vi "FRC Color Processing Example.vi"() -> ()   [LabVIEW 2019]
uses:
  <vilib>/Rock Robotics/WPI/Camera/WPI_CameraSettings Read MJPG.ctl
  <vilib>/Rock Robotics/WPI/Camera/WPI_CameraImageSize.ctl
  Vision Support Code/Camera Types.ctl
  <vilib>/Rock Robotics/WPI/Camera/WPI_CameraExposure Values.ctl
  <vilib>/Rock Robotics/WPI/Camera/WPI_CameraWhite Balance Values.ctl
  <vilib>/vision/NI_Vision_Development_Module.lvlib
panel:
  out "Number of Particles":i32
  out "Particle Measurements (Pixels)":dbl[][](array[numeric]) format="%.2f"
  out "Particle Measurements (Real-World)":dbl[][](array[numeric]) format="%.2f"
  in  "Min Compnt %":dbl=15.0
  out "Results":T1(array[cluster]) {"Score" format="%#_3g"; "Pixels"."Rectangle"."Numeric 5" format="%#_3g"; "Pixels"."Rectangle"."Numeric 3" format="%#_3g"; "Pixels"."Rectangle"."Numeric 2" format="%#_3g"; "Pixels"."Rectangle"."Numeric" format="%#_3g"; "Normalized"."Rectangle"."Numeric 5" format="%#_2g"; "Normalized"."Rectangle"."Numeric 3" format="%#_2g"; "Normalized"."Rectangle"."Numeric 2" format="%#_2g"; "Normalized"."Rectangle"."Numeric" format="%#_2g"; "Normalized"."Center"."?" format="%#_3g"; "Normalized"."Center"."?" format="%#_3g"; "Distance (ft)" format="%#_3g"}
  in  "Size Limit %":dbl=0.04 min=0.0 max=100.0 step=0.01 format="%#_13g"
  out "Instructions:":string="Instructions:\nUse Source to load image files from a directory, or use a USB or IP camera connected to your laptop. Use Camera Settings 1 and 2 to achieve a dark image with bright and colorful stripes.\nLED Color can encoded as HSL or related color modes. Calibrate to the same color as the strips being reflected to the camera.\nClick and draw a line in Original Image to auto-calibrate the LED Color. You may want to widen and tweak Sat and Val by hand.\nThe Annotate button affects drawing a rectangle around the stripes and labeling it with a distance in ft. Distance relies on knowing the Camera Type and lens calibration (it looks up the lens view angle).\n\nAdjust Score Cutoff to make the code more or less picky. If the color is not very unique, you may need to increase the number of particles considered. The diagram uses a Size Limit to ignore colored things that are too small. You may need to adjust it if you are targetting from far away.\n\nResults give you the distance to the target, the center and box in a normalized (-1 to 1) and pixel coordinates.\n\nBe sure to read about setting camera exposure and brightness to help simplify your image and acquire color saturated images.\n\nThere are lots of comments on the diagram to explain the code."
  in  "Color Mode":u16(ring)=2 items=["RGB", "HSL", "HSV", "HSI"]
  in  "Particles":dbl=5.0
  in  "Score Cutoff %":dbl=75.0
  in  "Std Devs for Calibration":cluster{"H":dbl, "S":dbl, "V":dbl}={"H"=4.0, "S"=8.0, "V"=8.0}
  in  "Camera Type (for distance)":T2=enum."MS HD3000 square"
  in  "image files":string[](array[string])
  in  "Source":enum32{"Files", "Camera"}(tab)
  in  "Images":i32(listbox)
  in  "Folder Location":path=path "C:/Program Files (x86)/National Instruments/LabVIEW 2018/examples/FRC/roboRIO/Vision/2019 Vision Example/Sample Images"
  in  "Camera Settings":T3={"fps"=20, "compression"=30, "Image Size"=enum."320x240", "Config Shown"=FALSE}
  in  "Camera Address":string="USB 1"
  in  "Camera Settings 2":T7={"Exposure"=enum."Auto", "Exposure (%)"=50.0, "Brightness"=50, "White Balance"=enum."Auto", "Color Temp (K)"=0.0} {"Brightness" min=0 max=100}
  in  "Annotate":bool=TRUE
  out "Qualified Particles":i32
  in  "LED Color Range":T8={"Hue"={75.46666717529297, 107.46666717529297}, "Sat"={221.18788146972656, 255.0}, "Val"={23.733230590820312, 172.13343811035156}} {"Hue" scale=0.0..255.0 scale format="%#_3g"}
  out "Mask":T9(plugin-control)
  out "Original Image":T9(plugin-control)
  # "Good target rectangle, distance ft"
  # "Bad target rectangle"
  # "Score in %"
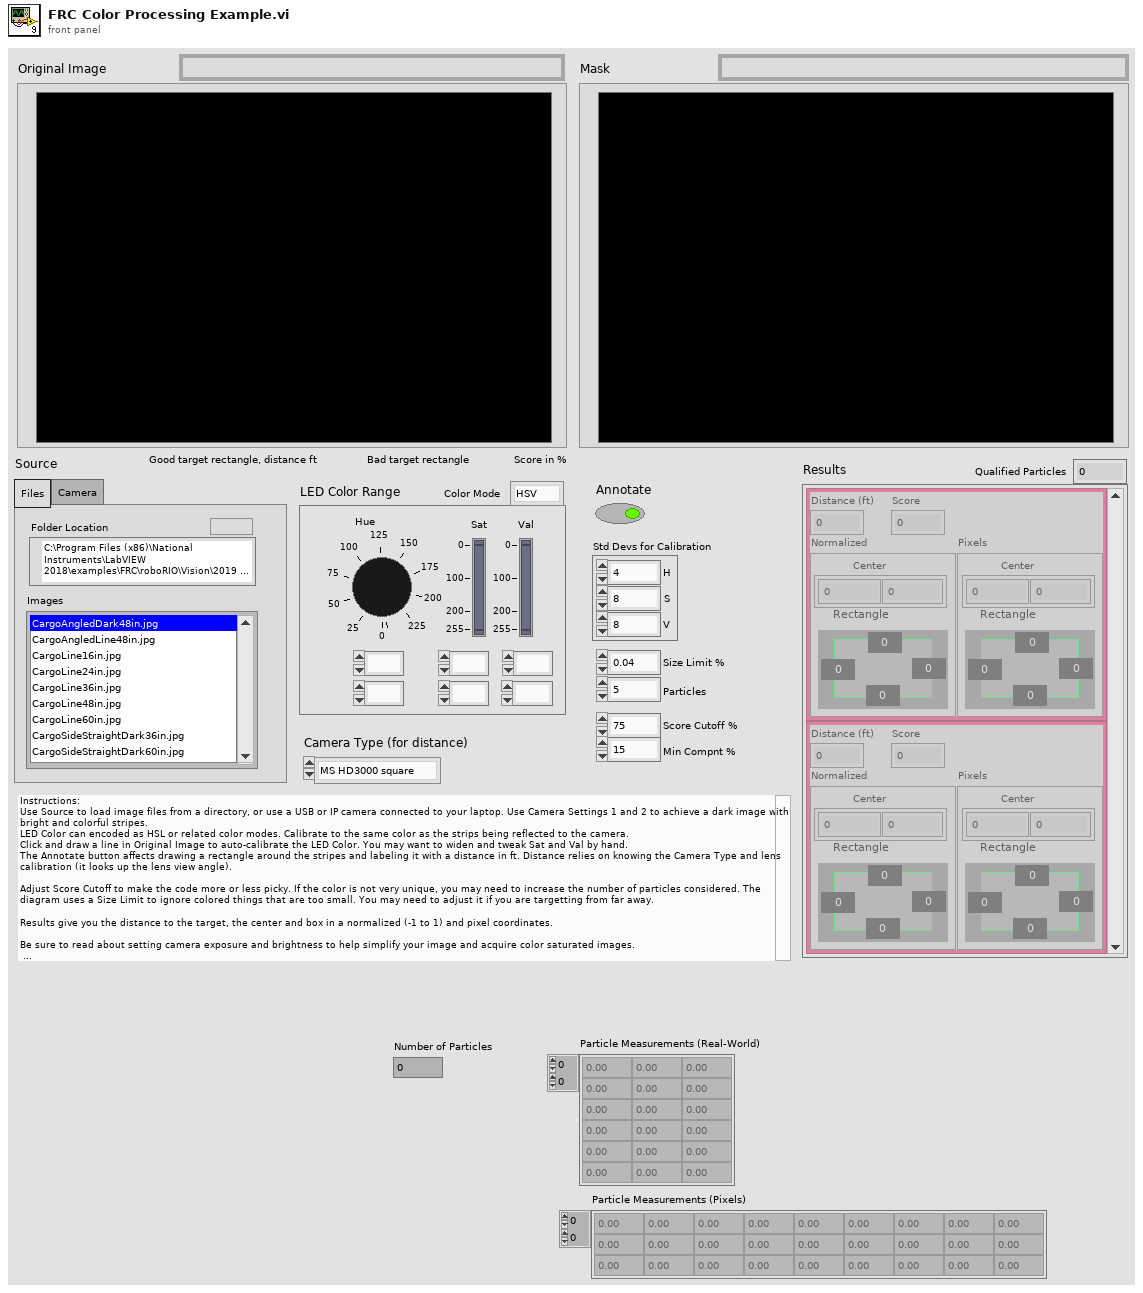
[diagram p1: front panel]
types:
  T1 = cluster{"Distance (ft)":dbl, "Score":dbl, "Normalized":cluster{"Center":cluster{dbl, dbl}, "Rectangle":cluster{"Numeric":dbl, "Numeric 2":dbl, "Numeric 3":dbl, "Numeric 5":dbl}}, "Pixels":cluster{"Center":cluster{dbl, dbl}, "Rectangle":cluster{"Numeric":dbl, "Numeric 2":dbl, "Numeric 3":dbl, "Numeric 5":dbl}}}[]
  T2 = typedef "Camera Types.ctl" = enum16{"206", "1011", "1013", "MS HD3000 square", "MS HD3000 640x480"}
  T3 = typedef "WPI_CameraSettings Read MJPG.ctl" = cluster{"fps":i32, "compression":i32, "Image Size":T4, "Config Shown":bool}
  T4 = typedef "WPI_CameraImageSize.ctl" = enum16{"640x480", "320x240", "160x120", "Custom"}
  T5 = typedef "WPI_CameraExposure Values.ctl" = enum16{"Auto", "Flicker-free 50 Hz", "Flicker-free 60 Hz", "Hold current", "Custom"}
  T6 = typedef "WPI_CameraWhite Balance Values.ctl" = enum16{"Auto", "Fixed indoor", "Fixed outdoor 1", "Fixed outdoor 2", "Fixed fluorescent 1", "Fixed fluorescent 2", "Hold current", "Custom"}
  T7 = cluster{"Exposure":T5, "Exposure (%)":dbl, "Brightness":i32, "White Balance":T6, "Color Temp (K)":dbl}
  T8 = cluster{"Hue":cluster{dbl, dbl}, "Sat":cluster{dbl, dbl}, "Val":cluster{dbl, dbl}}
  T9 = typedef "IMAQ Image.ctl" = refnum<image>
  T10 = typedef "Particle Parameters" = i32
  T11 = typedef "Image Type" = u32
  T12 = cluster{cluster{dbl, dbl}, cluster{dbl, dbl}, cluster{dbl, dbl}}
  T13 = cluster{"Score":dbl, "Rect":cluster{"Left":dbl, "Top":dbl, "Right":dbl, "Bottom":dbl}, "Full Scores":cluster{"Aspect Ratio":dbl, "Top Position":dbl, "Bottom Position":dbl, "Left Gap":dbl, "Width":dbl, "Height Ratio":dbl, "Angle":dbl}}[]
  T14 = cluster{"Left":dbl, "Top":dbl, "Right":dbl, "Bottom":dbl}
  T15 = cluster{"Distance (ft)":dbl, "Score":dbl, "Normalized":cluster{"Center":cluster{dbl, dbl}, "Rectangle":cluster{"Numeric":dbl, "Numeric 2":dbl, "Numeric 3":dbl, "Numeric 5":dbl}}, "Pixels":cluster{"Center":cluster{dbl, dbl}, "Rectangle":cluster{"Numeric":dbl, "Numeric 2":dbl, "Numeric 3":dbl, "Numeric 5":dbl}}}
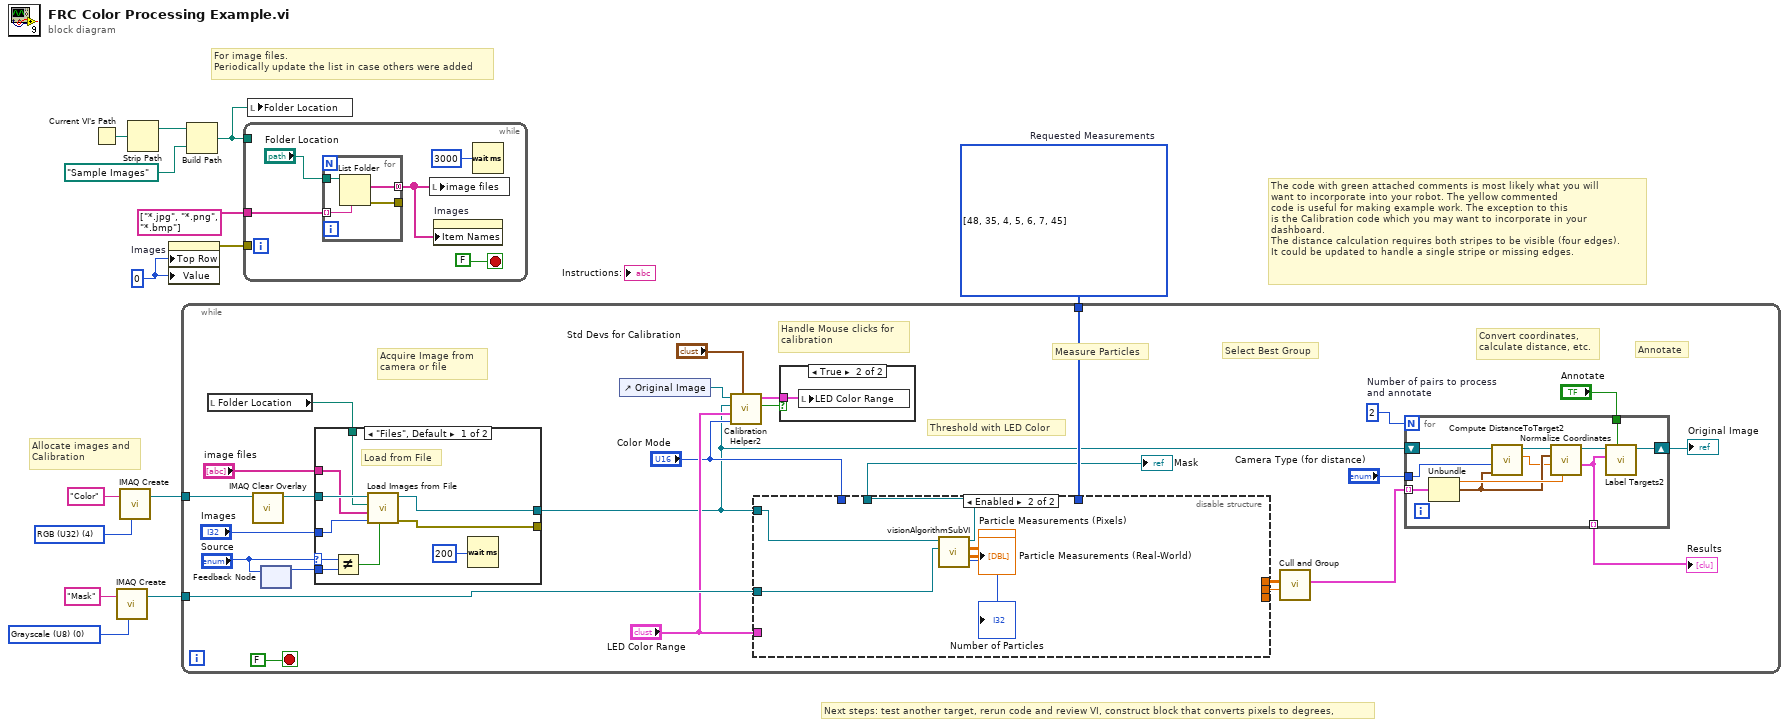
[diagram p0: block diagram]
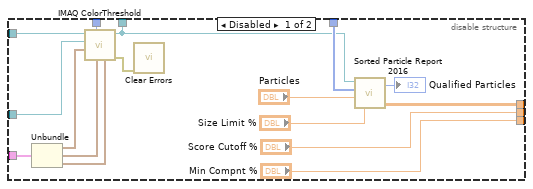
[diagram p2: hidden frame]
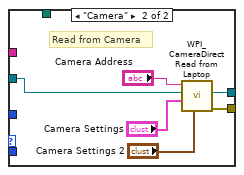
[diagram p4: hidden frame]
diagram:
  w3 = u32 0 ("milliseconds to wait")
  w9 = T10[] [48, 35, 4, 5, 6, 7, 45] items=["Center of Mass X", "Center of Mass Y", "First Pixel X", "First Pixel Y", "Bounding Rect Left", "Bounding Rect Top", "Bounding Rect Right", "Bounding Rect Bottom", "Max Feret Diameter Start X", "Max Feret Diameter Start Y", "Max Feret Diameter End X", "Max Feret Diameter End Y", "Max Horiz. Segment Length Left", "Max Horiz. Segment Length Right", "Max Horiz. Segment Length Row", "-", "Bounding Rect Width", "Bounding Rect Height", "Bounding Rect Diagonal", "Perimeter", "Convex Hull Perimeter", "Holes' Perimeter", "Max Feret Diameter", "Equivalent Ellipse Major Axis", "Equivalent Ellipse Minor Axis", "Equivalent Ellipse Minor Axis (Feret)", "Equivalent Rect Long Side", "Equivalent Rect Short Side", "Equivalent Rect Diagonal", "Equivalent Rect Short Side (Feret)", "Average Horiz. Segment Length", "Average Vert. Segment Length", "Hydraulic Radius", "Waddel Disk Diameter", "-", "Area", "Holes' Area", "Particle & Holes' Area", "Convex Hull Area", "Image Area", "-", "Number of Holes", "Number of Horiz. Segments", "Number of Vert. Segments", "-", "Orientation", "Max Feret Diameter Orientation", "-", "% Area/Image Area", "% Area/(Particle & Holes' Area)", "Ratio of Equivalent Ellipse Axes", "Ratio of Equivalent Rect Sides", "-", "Elongation Factor", "Compactness Factor", "Heywood Circularity Factor", "Type Factor", "-", "Sum X", "Sum Y", "Sum XX", "Sum XY", "Sum YY", "Sum XXX", "Sum XXY", "Sum XYY", "Sum YYY", "-", "Moment of Inertia XX", "Moment of Inertia XY", "Moment of Inertia YY", "Moment of Inertia XXX", "Moment of Inertia XXY", "Moment of Inertia XYY", "Moment of Inertia YYY", "Norm. Moment of Inertia XX", "Norm. Moment of Inertia XY", "Norm. Moment of Inertia YY", "Norm. Moment of Inertia XXX", "Norm. Moment of Inertia XXY", "Norm. Moment of Inertia XYY", "Norm. Moment of Inertia YYY", "Hu Moment 1", "Hu Moment 2", "Hu Moment 3", "Hu Moment 4", "Hu Moment 5", "Hu Moment 6", "Hu Moment 7"]  # Requested Measurements
  w12 = T11 0 items=["Grayscale (U8)", "Grayscale (I16)", "Grayscale (SGL)", "Complex (CSG)", "RGB (U32)", "HSL (U32)", "RGB (U64)", "Grayscale (U16)"] ("Image Type")
  w13 = T11 4 items=["Grayscale (U8)", "Grayscale (I16)", "Grayscale (SGL)", "Complex (CSG)", "RGB (U32)", "HSL (U32)", "RGB (U64)", "Grayscale (U16)"] ("Image Type")
  # "Next steps: test another target, rerun code and review VI, construct block that converts pixels to degrees,"
  # "The code with green attached comments is most likely what you will\nwant to incorporate into your robot. The yellow commented\ncode is useful for making example work. The exception to this\nis the Calibration code which you may want to incorporate in your\ndashboard.\nThe distance calculation requires both stripes to be visible (four edges).\nIt could be updated to handle a single stripe or missing edges."
  # "For image files.\nPeriodically update the list in case others were added"
  # "Allocate images and\nCalibration"
  n1 = Current VI's Path() -> (path=w8:path)
  n2 = call "IMAQ Create"("Image Name"="Mask", "Image Type"=w12) -> ("New Image"=w10:T9)  [unwired: 2 in, 2 out]
  n3 = call "IMAQ Create"("Image Name"="Color", "Image Type"=w13) -> ("New Image"=w1:T9)  [unwired: 2 in, 2 out]
  n4 = Strip Path(path=w8) -> (stripped path=w6:path)  [unwired: 1 out]
  n5 = property on="Images" class="LstBox (strict)"("Top Row"=w3, "Value"=w3) -> (error out=w4:errorcluster)  [unwired: 2 in, 1 out]
  n6 = while {
    tunnel: w1 -> [w20]
    tunnel: w10 -> [w38]
    tunnel: w9 -> [w37]
    stop <- FALSE stop-if-true
    w21 = 2  # Number of pairs to process and annotate
    # "Handle Mouse clicks for\ncalibration"
    # "Measure Particles"
    # "Convert coordinates,\ncalculate distance, etc."
    # "Annotate"
    # "Select Best Group"
    # "Threshold with LED Color"
    # "Acquire Image from\ncamera or file"
    n7 = local read "Folder Location"() -> (w30:path)
    n8 = call "IMAQ Clear Overlay"("Image"=w20) -> ("Image Out"=w19:T9)  [unwired: 2 in, 8 out]
    n9 = feedback-in #1("Source") -> ()
    n10 = feedback #1() -> (w28:enum32{"Files", "Camera"})  [unwired: 1 in]
    n11 = case shown="\"Files\", Default" "Source" {
      selector: "Source" -> [w77 _]
      tunnel: [w83 w90] -> _
      tunnel: [w84 w89] -> w17
      tunnel: w19 -> [w82 w88]
      tunnel: "image files" -> [w79 _]
      tunnel: "Images" -> [w81 _]
      tunnel: w30 -> [w80 _]
      tunnel: w28 -> [w76 _]
      frame "Files", Default {
        # "Load from File"
        n12 = Not Equal?(x=w77, y=w76) -> (x != y?=w75:bool)
        n13 = call "Load Images from File.vi"("Force Load"=w75, "Images"=w81, "image files"=w79, "Folder Location"=w80, "Refnum in"=w82) -> ("error out"=w83:errorcluster, "Refnum out"=w84:T9)  [unwired: 5 in]
        n14 = Wait (ms)(milliseconds to wait=u32 200 ("delay (ms)")) -> ()  [unwired: 1 out]
      }
      frame "Camera" {
        # "Read from Camera"
        n15 = call <vilib>:"WPI_CameraDirect Read from Laptop.vi"("Camera Settings 2"="Camera Settings 2", "Camera Settings"="Camera Settings", "Image"=w88, "address"="Camera Address") -> ("error out"=w90:errorcluster, "Image Out"=w89:T9)  [unwired: 6 in]
      }
    }
    n16 = control-ref of="Original Image"() -> (w35:refnum<vi>)
    n17 = call "Calibration Helper2.vi"("Std Devs"="Std Devs for Calibration", "Color Mode"="Color Mode", "Color Components"="LED Color Range", "Image"=w17, "Image Ctl Refnum"=w35) -> ("Changed"=w34:bool, "output color"=w33:T12)  [unwired: 5 in]
    n18 = disable-structure shown="Enabled" {
      disable-tunnel: w38 -> [w56 w60]
      disable-tunnel: w37 -> [w52 _]
      disable-tunnel: "LED Color Range" -> [w48 _]
      disable-tunnel: [w47 _] -> w15
      disable-tunnel: "Color Mode" -> [w45 _]
      disable-tunnel: ["Score Cutoff %" _] -> w23
      disable-tunnel: w17 -> [w43 w61]
      disable-tunnel: ["Min Compnt %" _] -> _
      disable-tunnel: [w41 w62] -> w16
      frame Disabled {
        n19 = Unbundle(w48) -> ("Hue"=w55:cluster{dbl, dbl}, "Sat"=w54:cluster{dbl, dbl}, "Val"=w53:cluster{dbl, dbl})
        n20 = call "IMAQ ColorThreshold"("Blue or Luma or Val or Inten Range"=w53, "Green or Sat Range"=w54, "Color Mode"=w45, "Red or Hue Range"=w55, "Image Dst"=w56, "Image Src"=w43) -> ("error out"=w49:errorcluster, "Image Dst Out"=w41:T9)  [unwired: 4 in]
        n21 = call <vilib>:"Clear Errors.vi"("error in (no error)"=w49) -> ()  [unwired: 5 in, 2 out]
        n22 = call "Sorted Particle Report 2016.vi"("Min Area Size %"="Size Limit %", "Particle Count Limit"="Particles", "Pixel Measurements"=w52, "Image in"=w41) -> ("Sorted Data"=w47:dbl[][], "Particles"=→"Qualified Particles":i32)
      }
      frame Enabled {
        n23 = call "visionAlgorithmSubVI.vi"("Image Dst"=w60, "Refnum in"=w61) -> ("Particle Measurements (Real-World)"=→"Particle Measurements (Real-World)":dbl[][], "Particle Measurements (Pixels)"=→"Particle Measurements (Pixels)":dbl[][], "Refnum out"=w62:T9, "Number of Particles"=→"Number of Particles":i32)  [unwired: 5 in, 1 out]
      }
    }
    "Mask" <- w16
    n24 = case shown="True" w34 {
      tunnel: w33 -> [_ w74]
      frame False {
      }
      frame True {
        n25 = local write "LED Color Range"(w74) -> ()
      }
    }
    n26 = call "Cull and Group.vi"("Score Cutoff %"=w23, "Sorted Data"=w15) -> ("Best Targets above cutoff"=w27:T13)  [unwired: 9 in]
    n27 = for {
      N: w21 -> [_]
      tunnel: [w72] -> w18 mode=indexing
      tunnel: w27 -> [w68] mode=indexing
      tunnel: "Camera Type (for distance)" -> [w71]
      tunnel: "Annotate" -> [w64]
      shift-right: [w69] -> w22
      shift-left: w17 -> [w70]
      n28 = Unbundle(w68) -> ("Score"=w67:dbl, "Rect"=w65:T14)  [unwired: 1 out]
      n29 = call "Compute DistanceToTarget2.vi"("Rect"=w65, "Camera Type"=w71, "Image Src"=w70) -> ("Distance (ft)"=w63:dbl, "Image Dst Out"=w66:T9)  [unwired: 7 in]
      n30 = call "Normalize Coordinates.vi"("Score"=w67, "Distance"=w63, "Bounding box"=w65, "Image in"=w66) -> ("Results"=w72:T15, "Image out"=w73:T9)  [unwired: 6 in]
      n31 = call "Label Targets2.vi"("Annotate"=w64, "Results"=w72, "Image in"=w73) -> ("Image out"=w69:T9)  [unwired: 8 in]
    }
    "Original Image" <- w22
    "Results" <- w18
  }
  n32 = Build Path(base path=w6, name or relative path=path "Sample Images" ("Folder Location")) -> (appended path=w5:path)
  n33 = while {
    tunnel: w5 -> [_]
    tunnel: w4 -> [_]
    tunnel: string[] ["*.jpg", "*.png", "*.bmp"] -> [w91]
    stop <- FALSE stop-if-true
    n34 = for {
      tunnel: [w99] -> w93 mode=concatenating
      tunnel: "Folder Location" -> [w98]
      tunnel: [w97] -> _
      tunnel: w91 -> [w96] mode=indexing
      n35 = List Folder(path=w98, pattern=w96) -> (filenames=w99:string[], error out=w97:errorcluster)  [unwired: 2 in, 2 out]
    }
    n36 = local write "image files"(w93) -> ()
    n37 = property on="Images" class="LstBox (strict)"("Item Names"=w93) -> ()  [unwired: 2 in, 2 out]
    n38 = Wait (ms)(milliseconds to wait=u32 3000) -> ()  [unwired: 1 out]
  }
  n39 = local write "Folder Location"(w5) -> ()
